vi "m1m3_acceptCommand_ApplyAberrationForces.vi"(8 "error in (no error)":errorcluster, 11 "command_ApplyAberrationForces_Ctl":T1) -> (0 "error out":errorcluster, 2 "function return":i32, 3 "command_ApplyAberrationForces_Ctl out":T1)   [LabVIEW 2016, in "SALLV_m1m3.lvlib"]
doc: "int m1m3_shm_acceptCommand_ApplyAberrationForcesLV(m1m3_command_ApplyAberrationForcesLV *command_ApplyAberrationForces_Ctl );"
uses:
  SALLV_m1m3.lvlib
  DataTypes/command_ApplyAberrationForces.ctl
  SALLV_m1m3.so
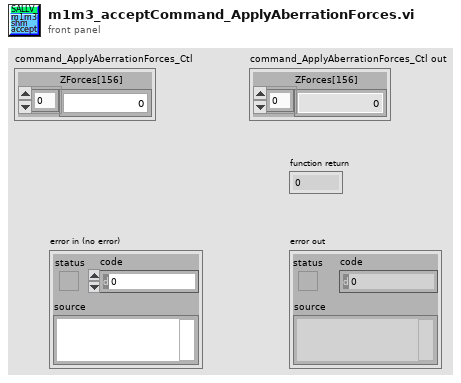
[diagram p1: front panel]
types:
  T1 = typedef "SALLV_m1m3.lvlib/command_ApplyAberrationForces.ctl" = cluster{"ZForces[156]":sgl[]}
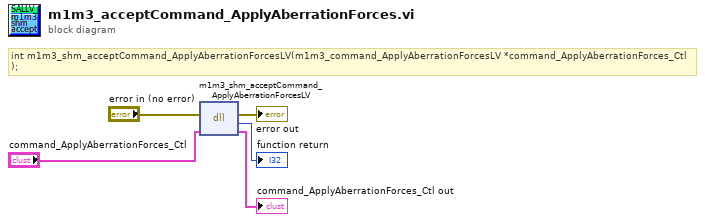
[diagram p0: block diagram]
diagram:
  # "int m1m3_shm_acceptCommand_ApplyAberrationForcesLV(m1m3_command_ApplyAberrationForcesLV *command_ApplyAberrationForces_Ctl );"
  n1 = dll-call lib="opt/CODE/SALLV_m1m3/SALLV_m1m3.*" fn="m1m3_shm_acceptCommand_ApplyAberrationForcesLV"(error in="error in (no error)", "command_ApplyAberrationForces_Ctl"="command_ApplyAberrationForces_Ctl") -> (error out=→"error out":errorcluster, →"function return":i32, "command_ApplyAberrationForces_Ctl"=→"command_ApplyAberrationForces_Ctl out":T1)  [unwired: 2 in, 1 out]
